vi "Hydrosonic_Conrol.vi"(2 "In range %":dbl format="%.2f", 3 "Input Mode":enum16{"Desired Frequency", "Transducer value"}(ring), 4 "Actual Sampling rate (Hz)":dbl=1000.0 format="%.2f", 5 "Desired Value":dbl format="%.2f") -> (0 "Error Info":string, 1 "Set output":dbl format="%.2f")   [LabVIEW 2012]
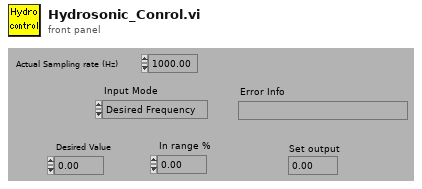
[diagram p1: front panel]
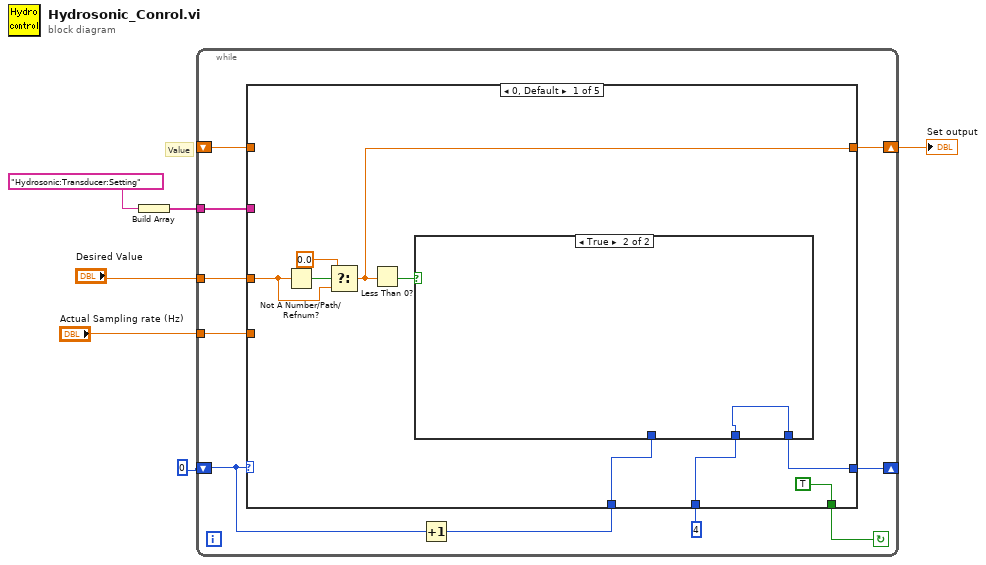
[diagram p0: block diagram]
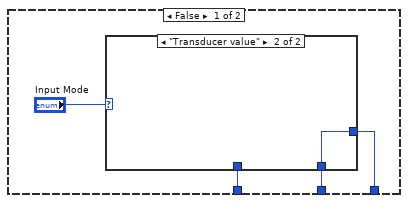
[diagram p2: hidden frame]
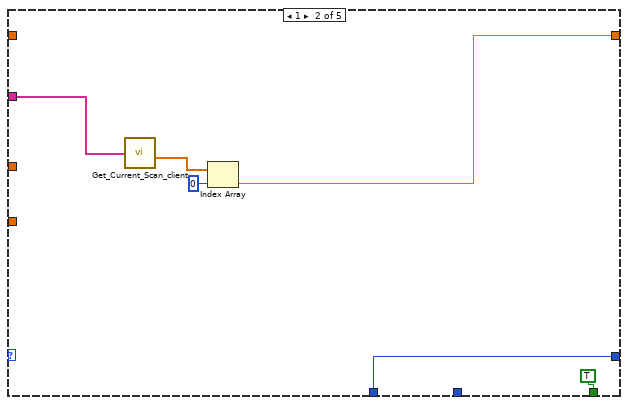
[diagram p4: hidden frame]
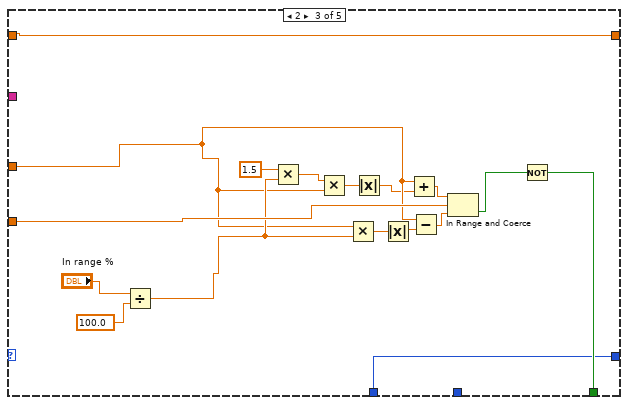
[diagram p5: hidden frame]
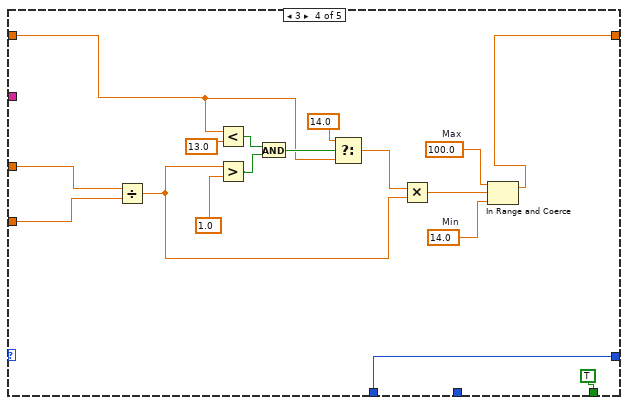
[diagram p6: hidden frame]
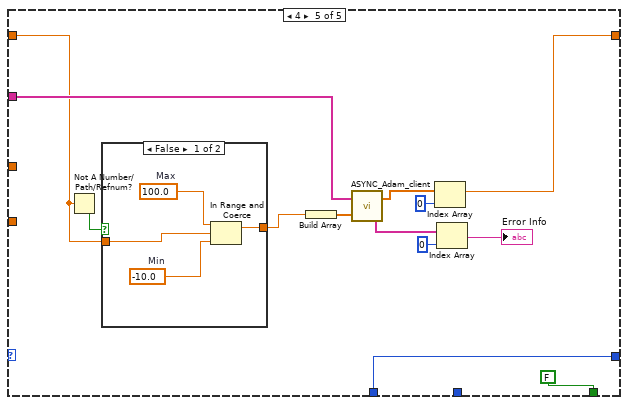
[diagram p7: hidden frame]
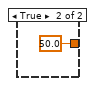
[diagram p8: hidden frame]
diagram:
  # "Value"
  n1 = Build Array("Hydrosonic:Transducer:Setting") -> (w3:string[])
  n2 = while {
    tunnel: "Actual Sampling rate (Hz)" -> [w9]
    tunnel: w3 -> [w11]
    shift-left: _ -> [w8]
    shift-right: [w10] -> w1
    tunnel: "Desired Value" -> [w16]
    shift-left: 0 -> [w15]
    shift-right: [w14] -> _
    stop <- w12 continue-if-true
    n3 = Increment(x=w15) -> (x+1=w13:i32)
    n4 = case shown="0, Default" w15 {
      tunnel: w16 -> [w20 _ w41 w70 _]
      tunnel: [w25 w34 w54 w72 w84] -> w14
      tunnel: w13 -> [w24 w34 w54 w72 w84]
      tunnel: [TRUE TRUE w55 TRUE FALSE] -> w12
      tunnel: w11 -> [_ w38 _ _ w78]
      tunnel: [w17 w35 w53 w56 w75] -> w10
      tunnel: w9 -> [_ _ w49 w69 _]
      tunnel: w8 -> [_ _ w53 w62 w73]
      tunnel: 4 -> [w22 _ _ _ _]
      frame 0, Default {
        n5 = Not A Number/Path/Refnum?(number/path/refnum=w20) -> (NaN/Path/Refnum?=w21:bool)
        n6 = Select(t=0.0, s=w21, f=w20) -> (s? t:f=w17:dbl)
        n7 = Less Than 0?(x=w17) -> (x < 0?=w18:bool)
        n8 = case shown="True" w18 {
          tunnel: [w28 w32] -> w25
          tunnel: w24 -> [w27 _]
          tunnel: w22 -> [w26 w32]
          frame False {
            n9 = case shown="\"Transducer value\"" "Input Mode" {
              tunnel: [w30 w31] -> w28
              tunnel: w27 -> [w30 _]
              tunnel: w26 -> [_ w31]
              frame "Desired Frequency" {
              }
              frame "Transducer value" {
              }
            }
          }
          frame True {
          }
        }
      }
      frame 1 {
        n10 = call "Get_Current_Scan_client.vi"("ADAM Ch Names"=w38) -> ("Numerical Values"=w37:dbl[])  [unwired: 3 out]
        n11 = Index Array(array=w37, index=0 ("Index")) -> (element=w35:dbl)
      }
      frame 2 {
        n12 = Divide(x="In range %", y=100.0) -> (x/y=w44:dbl)
        n13 = Multiply(x=1.5, y=w44) -> (x*y=w42:dbl)
        n14 = Multiply(x=w42, y=w41) -> (x*y=w43:dbl)
        n15 = Multiply(x=w41, y=w44) -> (x*y=w50:dbl)
        n16 = Absolute Value(x=w43) -> (abs(x)=w40:dbl)
        n17 = Absolute Value(x=w50) -> (abs(x)=w46:dbl)
        n18 = Add(x=w41, y=w40) -> (x+y=w52:dbl)
        n19 = Subtract(x=w41, y=w46) -> (x-y=w51:dbl)
        n20 = In Range and Coerce(upper limit=w52, x=w49, lower limit=w51) -> (In Range?=w39:bool)  [unwired: 1 out]
        n21 = Not(x=w39) -> (.not. x?=w55:bool)
      }
      frame 3 {
        w58 = 100.0  # Max
        w59 = 14.0  # Min
        n22 = Divide(x=w70, y=w69) -> (x/y=w60:dbl)
        n23 = Less?(x=w62, y=13.0) -> (x < y?=w65:bool)
        n24 = Greater?(x=w60, y=1.0) -> (0:w66:bool)
        n25 = And(x=w65, y=w66) -> (x .and. y?=w64:bool)
        n26 = Select(t=14.0, s=w64, f=w62) -> (s? t:f=w61:dbl)
        n27 = Multiply(x=w61, y=w60) -> (x*y=w57:dbl)
        n28 = In Range and Coerce(upper limit=w58, x=w57, lower limit=w59) -> (coerced(x)=w56:dbl)  [unwired: 1 out]
      }
      frame 4 {
        n29 = Not A Number/Path/Refnum?(number/path/refnum=w73) -> (NaN/Path/Refnum?=w74:bool)
        n30 = case shown="False" w74 {
          tunnel: w73 -> [w87 _]
          tunnel: [w86 50.0 ("Max")] -> w76
          frame False {
            w88 = 100.0  # Max
            w89 = -10.0  # Min
            n31 = In Range and Coerce(upper limit=w88, x=w87, lower limit=w89) -> (coerced(x)=w86:dbl)  [unwired: 1 out]
          }
          frame True {
          }
        }
        n32 = Build Array(w76) -> (w81:dbl[])
        n33 = call "ASYNC_Adam_client.vi"("Values"=w81, "Channel Names"=w78) -> ("Scan Comments"=w79:string[], "Calibrated Units"=w80:dbl[])
        n34 = Index Array(array=w80, index=0 ("Index")) -> (element=w75:dbl)
        n35 = Index Array(array=w79, index=0 ("Index")) -> (element=→"Error Info":string)
      }
    }
  }
  "Set output" <- w1
